vi "Evaluate Part 1.vi"() -> ()   [LabVIEW 2020]
uses:
  Schema Parser/Schema Parser.lvclass
  Number/Number.lvclass
panel:
  out "sum":i32=4361
  in  "String":string="467..114..\n...*......\n..35..633.\n......#...\n617*......\n.....+.58.\n..592.....\n......755.\n...$.*....\n.664.598.."
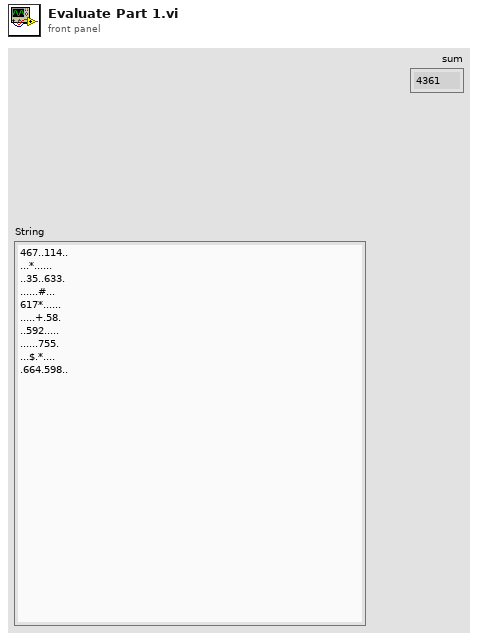
[diagram p1: front panel]
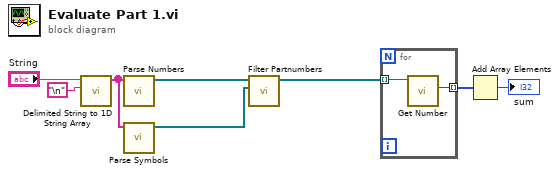
[diagram p0: block diagram]
diagram:
  n1 = call <vilib>:"Delimited String to 1D String Array.vi"("delimiter"="\n", "delimited string"="String") -> ("string array"=w6:string[])  [unwired: 9 in]
  n2 = call "Parse Numbers.vi"("string array"=w6) -> ("Array"=w5:refnum<class "Number.lvclass">[])  [unwired: 10 in]
  n3 = call "Parse Symbols.vi"("string array"=w6) -> ("Array"=w4:refnum<class "Symbol.lvclass">[])  [unwired: 10 in]
  n4 = call "Filter Partnumbers.vi"("Array in"=w4, "Array 3"=w5) -> ("Array out"=w3:refnum<class "Number.lvclass">[])  [unwired: 9 in]
  n5 = for {
    tunnel: w3 -> [w10] mode=indexing
    tunnel: [w9] -> w2 mode=indexing
    n6 = call "Get Number.vi"("Number in"=w10) -> ("Number"=w9:i32)  [unwired: 8 in, 2 out]
  }
  n7 = Add Array Elements(numeric array=w2) -> (sum=→"sum":i32)
